vi "Find All Devices.vi"(8 "error in (no error)":errorcluster) -> (0 "error out":errorcluster, 3 "Devices":refnum<class "Device.lvclass">[](array[class]))   [LabVIEW 2021, in "RTL-SDR.lvlib" / "Device.lvclass"]
uses:
  Device.lvclass
  Device.lvclass/Device.ctl
  lib/librtlsdr.dll
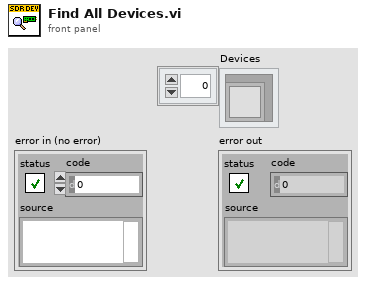
[diagram p1: front panel]
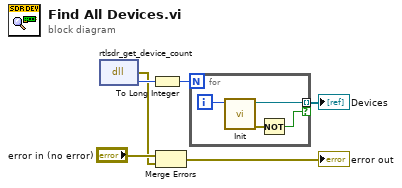
[diagram p0: block diagram]
diagram:
  n1 = dll-call lib="C:/dev/IlluminatedG/lv-rtl-sdr/lib/librtlsdr.dll" fn="rtlsdr_get_device_count"() -> (error out=w1:errorcluster, "return type"=w5:u32)  [unwired: 3 in, 1 out]
  n2 = To Long Integer(number=w5) -> (32bit integer=w4:i32)
  n3 = Merge Errors("error in (no error)", w1) -> (→"error out":errorcluster)
  n4 = for {
    N: w4 -> [_]
    tunnel: [w9] -> w3 mode=indexing if=w7
    i -> [w10]
    n5 = call "Init.vi"("Index"=w10) -> ("error out"=w8:errorcluster, "Device out"=w9:refnum<class "Device.lvclass">)  [unwired: 9 in]
    n6 = Not(x=w8) -> (.not. x?=w7:bool)
  }
  "Devices" <- w3
